vi "FTW-Test-SQLite-OpenCloseStress.vi"() -> (0 "Test Result":errorcluster)   [LabVIEW 2014]
uses:
  src/error/FTW-ERR-StatusOK.vi
  src/database/core/FTW-SQLite-Core-PrepareStatement.vi
  src/database/core/FTW-SQLite-Core-LibraryReturnValue.vi
  src/error/FTW-ERR-Assert-DeveloperError.vi
  src/database/core/FTW-SQLite-Core-QueryDebug.vi
  codegen/xnode/FTW-SQLite-Fetch.xnode
  src/database/core/FTW-SQLite-Core-Structure.ctl
panel:
  out "Result Set":T1(array[cluster])
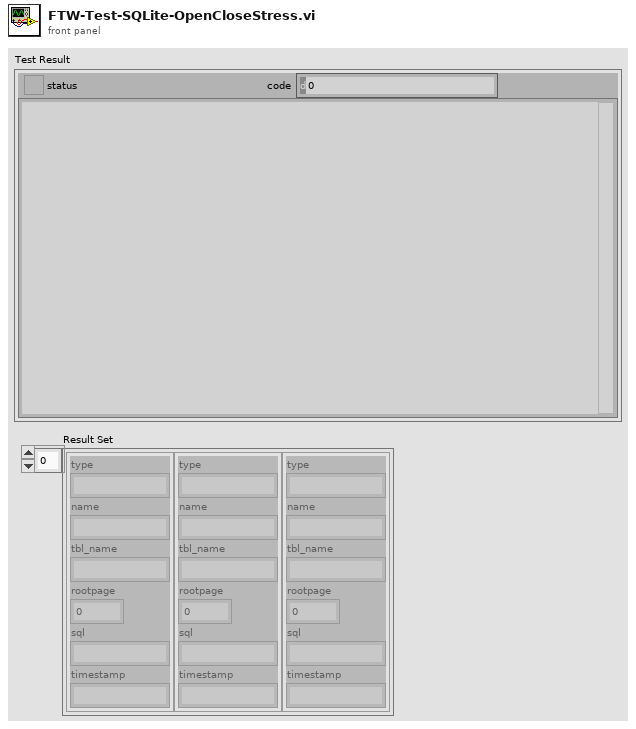
[diagram p1: front panel]
types:
  T1 = cluster{"type":string, "name":string, "tbl_name":string, "rootpage":i64, "sql":string, "timestamp":string}[]
  T2 = cluster{"type":string, "name":string, "tbl_name":string, "rootpage":i64, "sql":string, "timestamp":string}
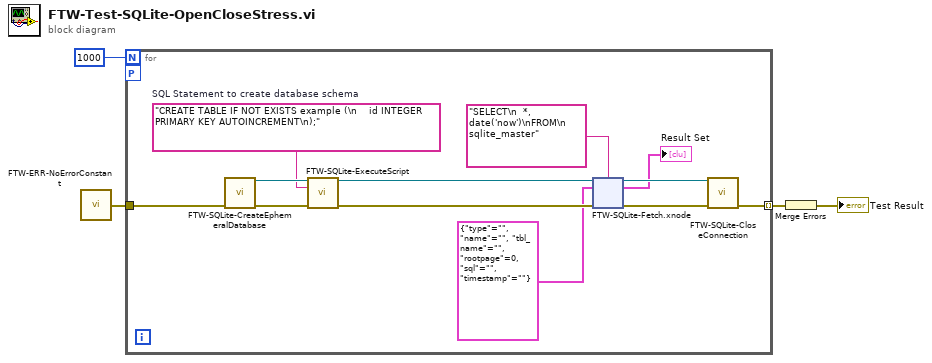
[diagram p0: block diagram]
diagram:
  n1 = call "FTW-ERR-NoErrorConstant.vi"() -> ("no error"=w1:errorcluster)
  n2 = for {
    N: 1000 -> [_]
    tunnel: [w13] -> w4 mode=indexing
    workers-P: _ -> [_]
    tunnel: w1 -> [w12]
    w14 = "CREATE TABLE IF NOT EXISTS example (\n    id INTEGER PRIMARY KEY AUTOINCREMENT\n);"  # SQL Statement to create database schema
    n3 = call "FTW-SQLite-CreateEphemeralDatabase.vi"("error in"=w12) -> ("SQLite Connection"=w15:refnum<data-value>, "error out"=w16:errorcluster)  [unwired: 13 in]
    n4 = call "FTW-SQLite-ExecuteScript.vi"("SQLite Connection"=w15, "SQL Script"=w14, "error in"=w16) -> ("SQLite Connection out"=w11:refnum<data-value>, "error out"=w9:errorcluster)  [unwired: 10 in, 1 out]
    n5 = xnode "FTW-SQLite-Fetch.xnode"("SQLite Connection"=w11, "SQL Script"="SELECT\n  *, date('now')\nFROM\n  sqlite_master", "Row Datatype"=T2 {"type"="", "name"="", "tbl_name"="", "rootpage"=0, "sql"="", "timestamp"=""}, "error in"=w9) -> ("SQLite Connection out"=w10:refnum<data-value>, "Result Set"=→"Result Set":T1, "error out"=w8:errorcluster)  [unwired: 1 out]
    n6 = call "FTW-SQLite-CloseConnection.vi"("SQLite Connection"=w10, "error in"=w8) -> ("error out"=w13:errorcluster)  [unwired: 13 in]
  }
  n7 = Merge Errors(w4) -> (→"Test Result":errorcluster)
